vi "Create Info Strings.vi"(5 "Include Secrets":bool, 6 "error in":errorcluster, 9 "Leaks":T1[](array[typedef])) -> (0 "error out":errorcluster, 3 "Info String":string)   [LabVIEW 2025]
doc: "This VI generates a string containing a short introduction, followed by a readable list of all detected secrets. Depending on the boolean input <b>Include Secrets</b>, the leaks will be explicitly added to the string.\n\nIf the <b>Leaks</b> Input is an empty string, this VI will generate a message to inform that no leaks were found."
uses:
  src/Type Definitions/Leak--cluster.ctl
  src/Type Definitions/Secret--cluster.ctl
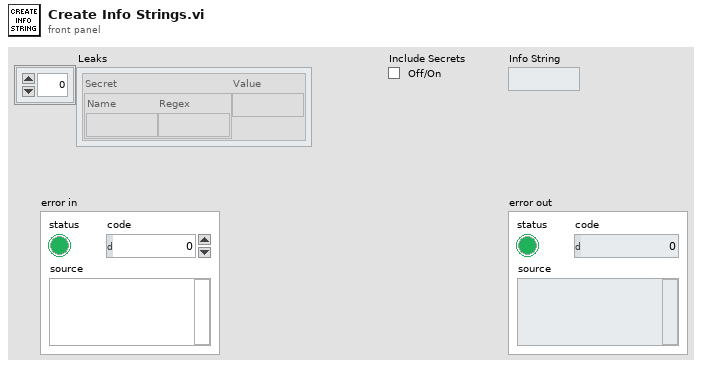
[diagram p1: front panel]
types:
  T1 = typedef "Leak--cluster.ctl" = cluster{"Secret":T2, "Value":string}
  T2 = typedef "Secret--cluster.ctl" = cluster{"Name":string, "Regex":string}
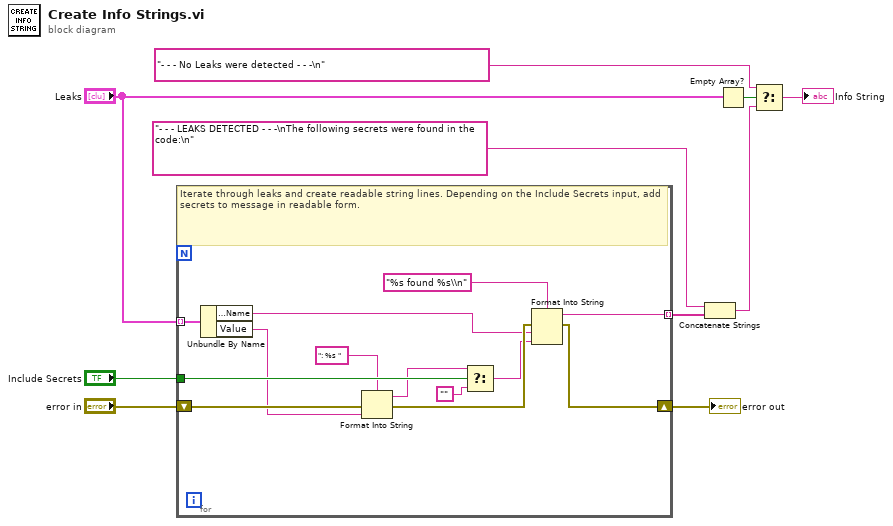
[diagram p0: block diagram]
diagram:
  n1 = for {
    tunnel: "Leaks" -> [w20] mode=indexing
    shift-right: [w23] -> w9
    shift-left: "error in" -> [w22]
    tunnel: "Include Secrets" -> [w17]
    tunnel: [w12] -> w8 mode=indexing
    # "Iterate through leaks and create readable string lines. Depending on the Include Secrets input, add secrets to message in readable form."
    n2 = Unbundle By Name(w20) -> ("Secret.Name"=w18:string, "Value"=w13:string)
    n3 = Format Into String(format string=": %s ", error in=w22, w13) -> (resulting string=w14:string, error out=w21:errorcluster)  [unwired: 1 in]
    n4 = Select(t=w14, s=w17, f="") -> (s? t:f=w11:string)
    n5 = Format Into String(format string="%s found %s\\n", error in=w21, w18, w11) -> (resulting string=w12:string, error out=w23:errorcluster)  [unwired: 1 in]
  }
  "error out" <- w9
  n6 = Concatenate Strings("- - - LEAKS DETECTED - - -\nThe following secrets were found in the code:\n", w8) -> (w2:string)
  n7 = Empty Array?(array="Leaks") -> (empty?=w4:bool)
  n8 = Select(t="- - - No Leaks were detected - - -\n", s=w4, f=w2) -> (s? t:f=→"Info String":string)
